vi "Flatten SocketCAN Header.vi"(8 "error in (no error)":errorcluster, 9 "Flattened Data in":u8[](array[numeric])=[0, 0, 0, 0, 0, 0, 0, 0] format="%.0x", 10 "CAN Header in":T1 {"CANID and Flags" format="%.0x"; "FD Flags" format="%.0x"}, 11 "pcap Parse and Build in":refnum<class "pcap_Parse_Build_CIF.lvclass">) -> (0 "error out":errorcluster, 1 "Flattened Data out":u8[](array[numeric])=[0, 0, 0, 0, 0, 0, 0, 0, 1, 2, 3, 4, 5], 2 "CAN Header out":T1 {"CANID and Flags" format="%.0x"; "FD Flags" format="%.0x"}, 3 "pcap Parse and Build out":refnum<class "pcap_Parse_Build_CIF.lvclass">)   [LabVIEW 2021, in "pcap_Parse_Build_CIF.lvclass"]
uses:
  pcap_Parse_Build_CIF.lvclass
  Typedef/Socket CAN Header.ctl
  pcap_Parse_Build_CIF.lvclass/pcap_Parse_Build_CIF.ctl
  e4177ba7-55c0-4140-bea2-15e5e44a53d0.vi
  e4177ba7-55c0-4140-bea2-15e5e44a53d0.vi/c28b0ead-42ad-4072-80a2-aca7f2bd7ce3.vi
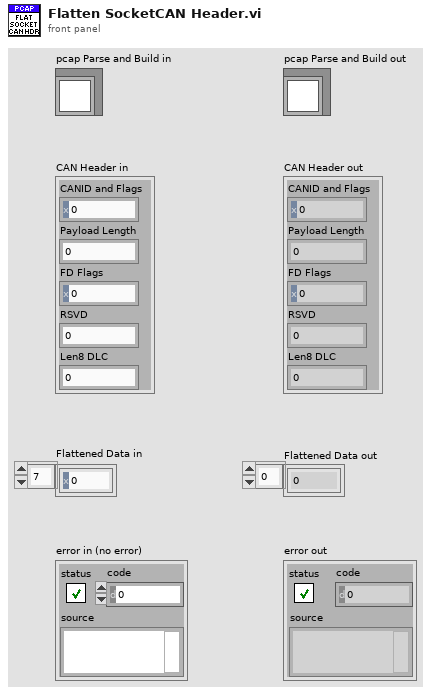
[diagram p1: front panel]
types:
  T1 = typedef "pcap_Parse_Build_CIF.lvclass/Socket CAN Header.ctl" = cluster{"CANID and Flags":u32, "Payload Length":u8, "FD Flags":u8, "RSVD":u8, "Len8 DLC":u8}
  T2 = typedef "DataTypes_CIF_U.lvlib/Endian.ctl" = enum16{"Little Endian", "Big Endian"}
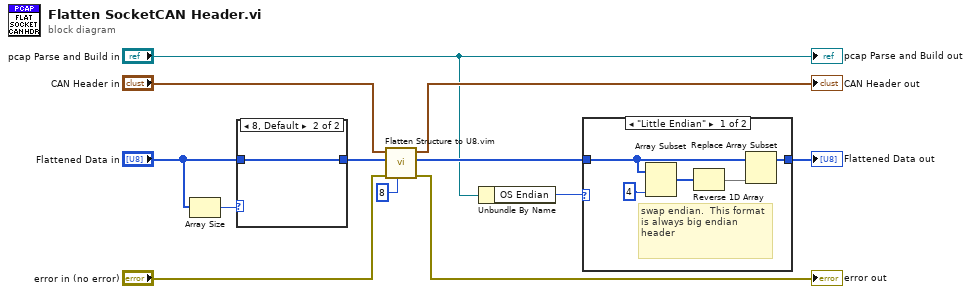
[diagram p0: block diagram]
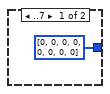
[diagram p3: hidden frame]
diagram:
  n1 = Array Size(array="Flattened Data in") -> (size(s)=w8:i32)
  n2 = case shown="8, Default" w8 {
    tunnel: "Flattened Data in" -> [_ w14]
    tunnel: [u8[] [0, 0, 0, 0, 0, 0, 0, 0] ("Flattened Data in") w14] -> w9
    frame ..7 {
    }
    frame 8, Default {
    }
  }
  n3 = call "Flatten Structure to U8.vim"("Length override"=u64 8, "error in"="error in (no error)", "Flattened Data in"=w9, "Data to Flatten in"="CAN Header in") -> ("error out"=→"error out":errorcluster, "Flattened Data out"=w7:u8[], "Data to Flatten out"=→"CAN Header out":T1)  [unwired: 5 in]
  n4 = Unbundle By Name("pcap Parse and Build in") -> ("OS Endian"=w1:T2)
  n5 = case shown="\"Little Endian\"" w1 {
    tunnel: w7 -> [w17 w20]
    tunnel: [w15 w20] -> w6
    frame "Little Endian" {
      # "swap endian.  This format is always big endian header"
      n6 = Array Subset(array=w17, length=4 ("index")) -> (w18:u8[])  [unwired: 1 in]
      n7 = Reverse 1D Array(array=w18) -> (reversed array=w16:u8[])
      n8 = Replace Array Subset(array=w17, new element=w16) -> (w15:u8[])  [unwired: 1 in]
    }
    frame "Big Endian" {
    }
  }
  "Flattened Data out" <- w6
  "pcap Parse and Build out" <- "pcap Parse and Build in"
